vi "SignalGenerator.vi"(1 "error in (no error)":errorcluster, 2 "Amplitude":dbl, 3 "Frequency":dbl) -> (0 "error out":errorcluster)   [LabVIEW 2015]
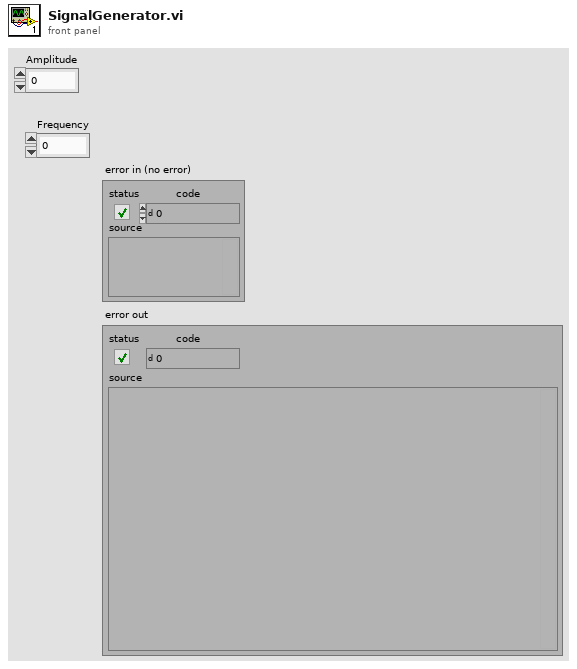
[diagram p1: front panel]
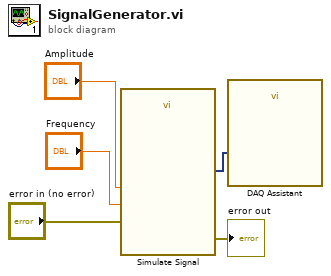
[diagram p0: block diagram]
diagram:
  n1 = call "Simulate Signal"("Frequency"="Frequency", "Amplitude"="Amplitude", "error in (no error)"="error in (no error)") -> ("Sine"=w3:dynamicdata, "error out"=→"error out":errorcluster)  [unwired: 11 in]
  n2 = call "DAQ Assistant"("data"=w3) -> ()  [unwired: 17 in, 2 out]
